vi "Constants.vi"() -> ()   [LabVIEW 2016, in "UDP Transmit Shared.lvlib"]
doc: "Use this Global VI to access the GUIDs assigned to the page resources of the Custom Device."
uses:
  UDP Transmit Shared.lvlib
panel:
  in  "Tab Control":enum32{"GUIDS", "Constants", "Properties"}(tab)
  in  "UDP Transmit":string="4494c228-26ed-4eb6-99bc-0aeb283ac215"
  in  "Destination Port":string
  in  "Destination IP Address":string
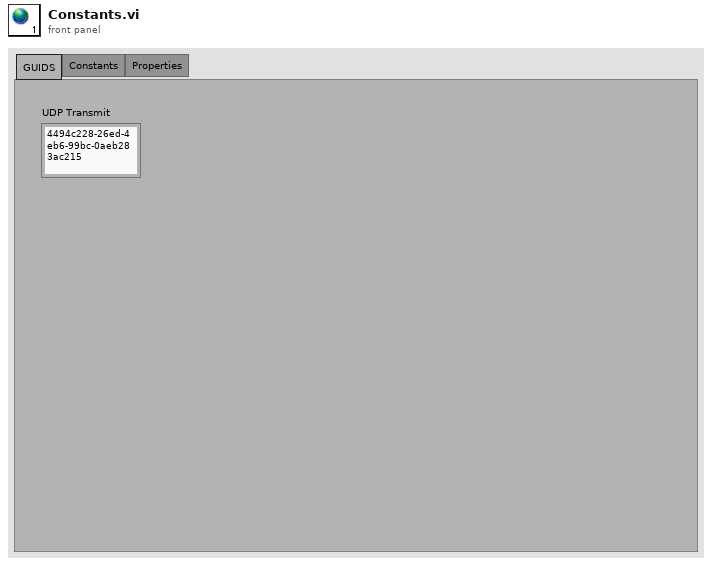
[diagram p1: front panel]
diagram:
